vi "Sensors - Convertion Calculation.vi"(0 "Input Value":dbl format="%.4f", 5 "Sensor type":T1, 7 "Translate To":T2, 9 "Input Table":dbl[][](array[numeric]) format="%.4f") -> (4 "Output Value":dbl format="%.4f", 15 "Error Out":errorcluster)   [LabVIEW 2011]
uses:
  Sensors - Controls/Sensors - Translation Type.ctl
  Sensors - Controls/Sensors - Temperature Sensor Type.ctl
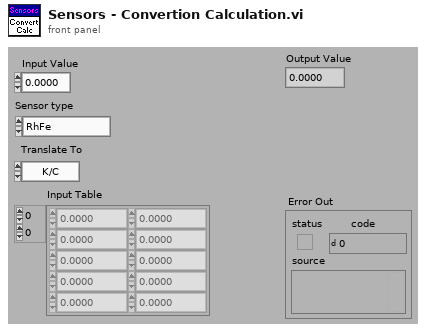
[diagram p1: front panel]
types:
  T1 = typedef "Sensors - Temperature Sensor Type.ctl" = enum16{"RhFe", "Pt", "K type thermocouple", "W5 type thermocouple", "No Conversion"}
  T2 = typedef "Sensors - Translation Type.ctl" = enum16{"K/C", "mV"}
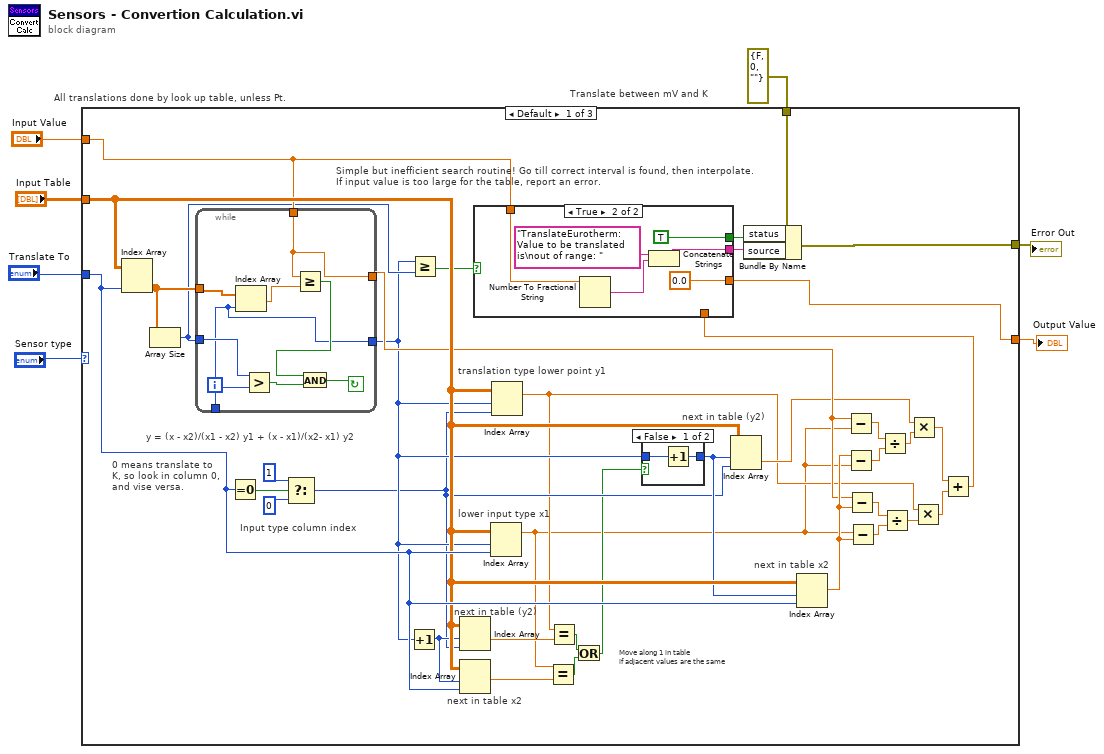
[diagram p0: block diagram]
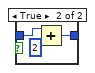
[diagram p2: hidden frame]
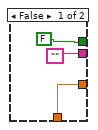
[diagram p3: hidden frame]
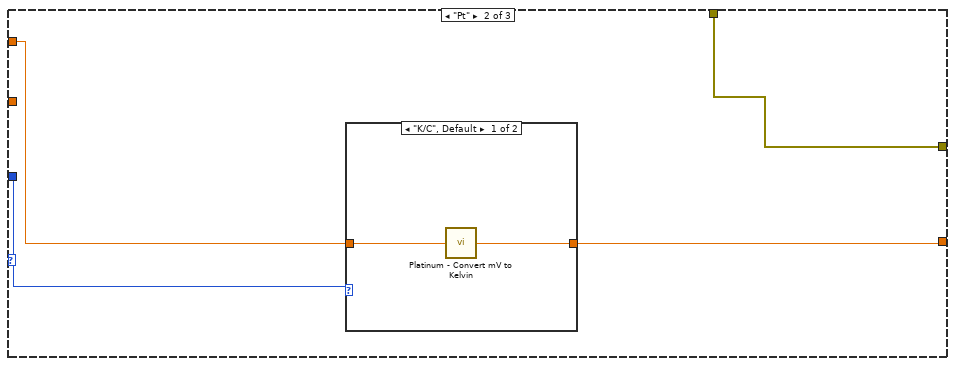
[diagram p4: hidden frame]
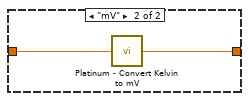
[diagram p5: hidden frame]
diagram:
  # "All translations done by look up table, unless Pt."
  # "Translate between mV and K"
  n1 = case shown="Default" "Sensor type" {
    tunnel: "Translate To" -> [w44 w70 _]
    tunnel: "Input Value" -> [w39 w69 w76]
    tunnel: "Input Table" -> [w43 _ _]
    tunnel: [w41 w68 w76] -> w5
    tunnel: errorcluster {"status"=FALSE, "code"=0, "source"=""} ("Error Out") -> [w40 w67 w75]
    tunnel: [w42 w67 w75] -> w4
    frame Default {
      # "next in table x2"
      # "next in table (y2)"
      # "Move along 1 in table\nif adjacent values are the same"
      # "next in table x2"
      # "lower input type x1"
      # "Input type column index"
      # "y = (x - x2)/(x1 - x2) y1 + (x - x1)/(x2- x1) y2"
      # "next in table (y2)"
      # "translation type lower point y1"
      # "Simple but inefficient search routine! Go till correct interval is found, then interpolate.\nIf input value is too large for the table, report an error."
      # "0 means translate to\nK, so look in column 0,\nand vise versa."
      n2 = Index Array(array=w43, index (col)=w44) -> (element=w35:dbl[])  [unwired: 1 in]
      n3 = Array Size(array=w35) -> (size(s)=w33:i32)
      n4 = while {
        tunnel: w35 -> [w66]
        tunnel: [w60] -> w17
        tunnel: [w59] -> w26
        tunnel: w33 -> [w61]
        tunnel: [w60] -> _
        tunnel: w39 -> [w59]
        i -> [w60]
        stop <- w62 continue-if-true
        n5 = Index Array(array=w66, index=w60) -> (element=w65:dbl)
        n6 = Greater?(x=w61, y=w60) -> (0:w64:bool)
        n7 = Greater Or Equal?(x=w59, y=w65) -> (x >= y?=w63:bool)
        n8 = And(x=w63, y=w64) -> (x .and. y?=w62:bool)
      }
      n9 = Equal To 0?(x=w44) -> (x = 0?=w37:bool)
      n10 = Select(t=1, s=w37, f=0) -> (s? t:f=w15:i32)
      n11 = Increment(x=w17) -> (x+1=w16:i32)
      n12 = Greater Or Equal?(x=w17, y=w33) -> (x >= y?=w34:bool)
      n13 = Index Array(array=w43, index (row)=w16, index (col)=w15) -> (element=w13:dbl)
      n14 = Index Array(array=w43, index (row)=w16, index (col)=w44) -> (element=w11:dbl)
      n15 = Index Array(array=w43, index (row)=w17, index (col)=w44) -> (element=w8:dbl)
      n16 = Index Array(array=w43, index (row)=w17, index (col)=w15) -> (element=w14:dbl)
      n17 = Equal?(x=w8, y=w11) -> (x = y?=w10:bool)
      n18 = Equal?(x=w14, y=w13) -> (x = y?=w12:bool)
      n19 = Or(x=w12, y=w10) -> (x .or. y?=w9:bool)
      n20 = case shown="False" w9 {
        tunnel: [w46 w49] -> w32
        tunnel: w17 -> [w45 w48]
        frame False {
          n21 = Increment(x=w45) -> (x+1=w46:i32)
        }
        frame True {
          n22 = Add(x=w48, y=2) -> (x+y=w49:i32)
        }
      }
      n23 = Index Array(array=w43, index (row)=w32, index (col)=w15) -> (element=w22:dbl)
      n24 = Index Array(array=w43, index (row)=w32, index (col)=w44) -> (element=w27:dbl)
      n25 = Subtract(x=w26, y=w8) -> (x-y=w25:dbl)
      n26 = Subtract(x=w27, y=w8) -> (x-y=w24:dbl)
      n27 = Subtract(x=w26, y=w27) -> (x-y=w31:dbl)
      n28 = Subtract(x=w8, y=w27) -> (x-y=w30:dbl)
      n29 = Divide(x=w25, y=w24) -> (x/y=w23:dbl)
      n30 = Divide(x=w31, y=w30) -> (x/y=w29:dbl)
      n31 = Multiply(x=w22, y=w23) -> (x*y=w21:dbl)
      n32 = Multiply(x=w14, y=w29) -> (x*y=w28:dbl)
      n33 = Add(x=w21, y=w28) -> (x+y=w18:dbl)
      n34 = case shown="True" w34 {
        tunnel: [FALSE TRUE] -> w20
        tunnel: ["" w53] -> w19
        tunnel: w18 -> [w50 _]
        tunnel: [w50 0.0] -> w41
        tunnel: w39 -> [_ w55]
        frame False {
        }
        frame True {
          n35 = Number To Fractional String(number=w55) -> (F-format string=w54:string)  [unwired: 3 in]
          n36 = Concatenate Strings("TranslateEurotherm: Value to be translated is\nout of range: ", w54) -> (w53:string)
        }
      }
      n37 = Bundle By Name(cluster=w40, "status"=w20, "source"=w19) -> (w42:errorcluster)
    }
    frame "Pt" {
      n38 = case shown="\"K/C\", Default" w70 {
        tunnel: w69 -> [w72 w74]
        tunnel: [w71 w73] -> w68
        frame "K/C", Default {
          n39 = call "Platinum - Convert mV to Kelvin.vi"("Platinum mV"=w72) -> ("Platinum K"=w71:dbl)  [unwired: 14 in]
        }
        frame "mV" {
          n40 = call "Platinum - Convert Kelvin to mV.vi"("Platinum K"=w74) -> ("Platinum mV"=w73:dbl)  [unwired: 14 in]
        }
      }
    }
    frame "No Conversion" {
    }
  }
  "Output Value" <- w5
  "Error Out" <- w4
